vi "to_json.vi"(8 "error in":errorcluster, 11 "target in":refnum<class "target.lvclass">) -> (0 "error out":errorcluster, 2 "json":string, 3 "target out":refnum<class "target.lvclass">, 4 "Not Default":bool)   [LabVIEW 2020, in "datasources.lvlib" / "target.lvclass"]
uses:
  target.lvclass
  target.lvclass/target.ctl
  dataset/dataset.lvclass/dataset.ctl
  92ef1fda-d962-45ff-88fd-c2047d5c0ec4.vi
  9fa72010-cb42-47d4-8643-e7e5955f5446.vi
  d6cf4258-1369-4a0e-93db-dcab189557e5.vi
  b2c1eefe-8312-4a03-882f-d0c7cc634c10.vi
  dataset/datasetName.get.vi
  dataset/datasetDescription.get.vi
  dataset/rid.get.vi
  <vilib>/JDP Science/JSONtext/Variant to JSON Text.vi
  <vilib>/JDP Science/JSONtext/support/Format JSON Object.vi
  <vilib>/JDP Science/JSONtext/LVClass Serializer/JSONtext LVClass Serializer.lvclass
  nominal types/properties/properties.lvclass
  nominal types/labels/labels.lvclass
  nominal types/channelConfig/channelConfig.lvclass
  nominal types/workspace/workspace.lvclass
  <vilib>/JDP Science/JSONtext/JSONtext.lvlib
  dataset/dataset.lvclass
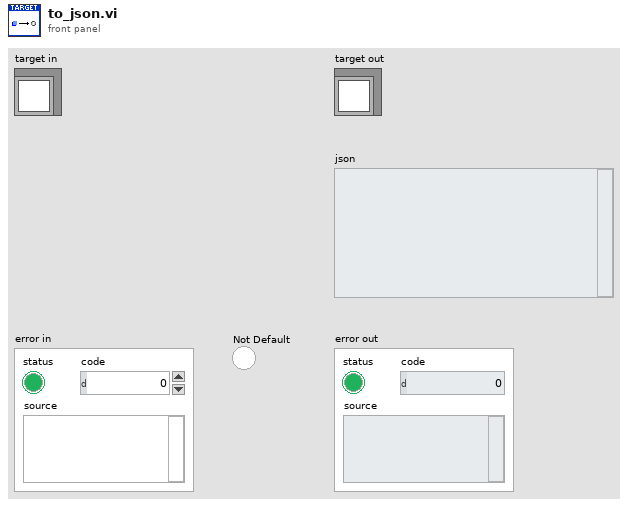
[diagram p1: front panel]
types:
  T1 = cluster{"type":string, "existing":cluster{"datasetRid":string}}
  T2 = cluster{"Accessors:datasetName":string, "Accessors:datasetDescription":string}
  T3 = cluster{"Accessors:datasetName":bool, "Accessors:datasetDescription":bool}
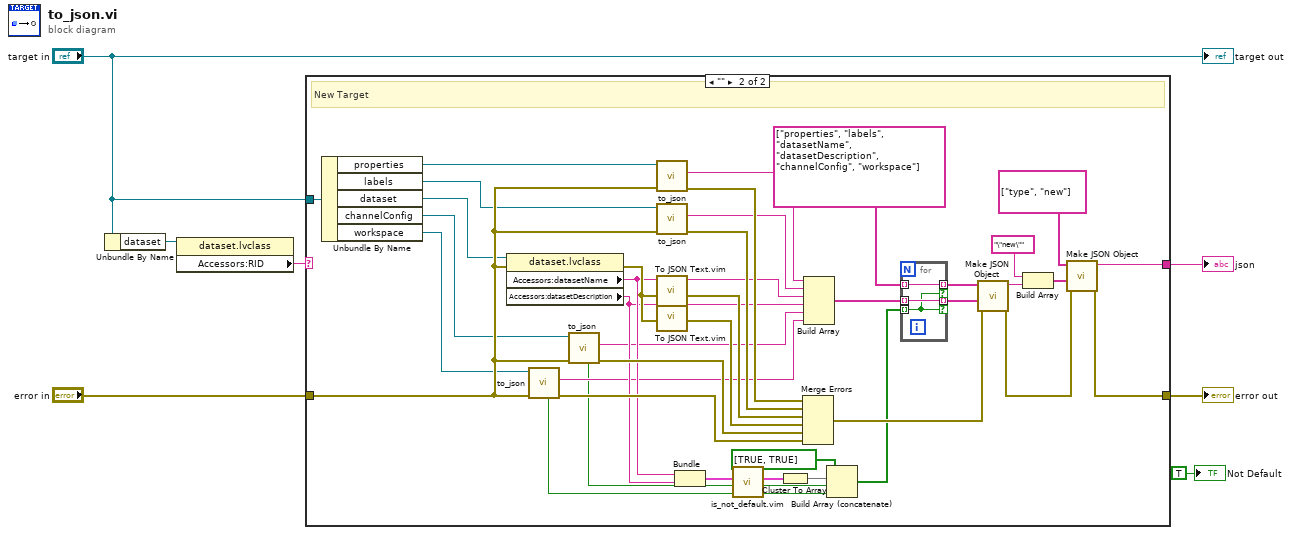
[diagram p0: block diagram]
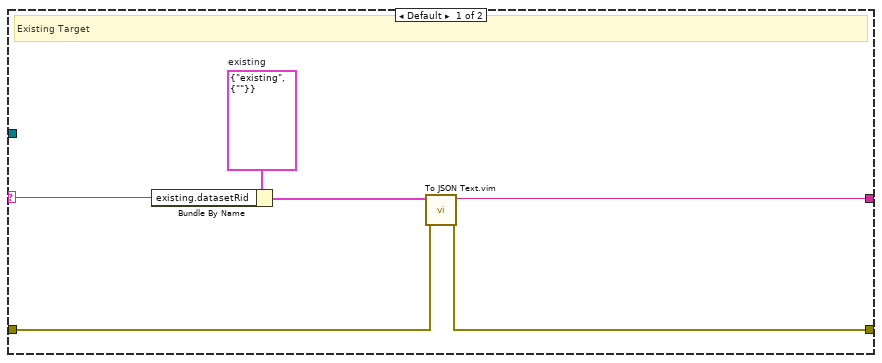
[diagram p2: hidden frame]
diagram:
  n1 = Unbundle By Name("target in") -> ("dataset"=w3:refnum<class "dataset.lvclass">)
  n2 = property class="dataset.lvclass"(reference=w3) -> ("Accessors:RID"=w2:string)  [unwired: 1 in, 2 out]
  n3 = case shown="\"\"" w2 {
    selector: w2 -> [w12 _]
    tunnel: [w10 w34] -> w7
    tunnel: "error in" -> [w9 w53]
    tunnel: [w8 w32] -> w5
    tunnel: "target in" -> [_ w47]
    frame Default {
      w13 = T1 {"type"="existing", "existing"={"datasetRid"=""}}  # existing
      # "Existing Target"
      n4 = Bundle By Name(cluster=w13, "existing.datasetRid"=w12) -> (w11:T1)
      n5 = call "To JSON Text.vim"("error in (no error)"=w9, "Anything"=w11) -> ("error out"=w8:errorcluster, "<JSON>"=w10:string)  [unwired: 8 in]
    }
    frame "" {
      # "New Target"
      n6 = Unbundle By Name(w47) -> ("properties"=w46:refnum<class "properties.lvclass">, "labels"=w45:refnum<class "labels.lvclass">, "dataset"=w27:refnum<class "dataset.lvclass">, "channelConfig"=w26:refnum<class "channelConfig.lvclass">, "workspace"=w25:refnum<class "workspace.lvclass">)
      n7 = property class="dataset.lvclass"(reference=w27, error in=w53) -> (error out=w54:errorcluster, "Accessors:datasetName"=w19:string, "Accessors:datasetDescription"=w18:string)  [unwired: 1 out]
      n8 = call-dynamic "to_json.vi"("error in"=w53, "workspace in"=w25) -> ("error out"=w40:errorcluster, "json"=w16:string, "Not Default"=w14:bool)  [unwired: 6 in, 1 out]
      n9 = call-dynamic "to_json.vi"("error in"=w53, "channelConfig in"=w26) -> ("error out"=w48:errorcluster, "json"=w17:string, "Not Default"=w15:bool)  [unwired: 6 in, 1 out]
      n10 = call-dynamic "to_json.vi"("error in"=w53, "properties in"=w46) -> ("error out"=w52:errorcluster, "json"=w44:string)  [unwired: 6 in, 2 out]
      n11 = call-dynamic "to_json.vi"("error in"=w53, "labels in"=w45) -> ("error out"=w51:errorcluster, "json"=w43:string)  [unwired: 6 in, 2 out]
      n12 = call "To JSON Text.vim"("error in (no error)"=w54, "Anything"=w19) -> ("error out"=w50:errorcluster, "<JSON>"=w42:string)  [unwired: 8 in]
      n13 = call "To JSON Text.vim"("error in (no error)"=w54, "Anything"=w18) -> ("error out"=w49:errorcluster, "<JSON>"=w41:string)  [unwired: 8 in]
      n14 = Bundle("Accessors:datasetName"=w19, "Accessors:datasetDescription"=w18) -> (w24:T2)  [unwired: 1 in]
      n15 = call "is_not_default.vim"("data"=w24) -> ("Not Default"=w23:T3)  [unwired: 10 in]
      n16 = Cluster To Array(cluster=w23) -> (array=w22:bool[])
      n17 = Merge Errors(w52, w51, w50, w49, w48, w40) -> (w39:errorcluster)
      n18 = Build Array(w44, w43, w42, w41, w17, w16) -> (w31:string[])
      n19 = Build Array (concatenate)(bool[] [TRUE, TRUE] ("element"), w22, w15, w14) -> (w20:bool[])
      n20 = for {
        tunnel: w31 -> [w57] mode=indexing
        tunnel: [w57] -> w30 mode=indexing if=w55
        tunnel: string[] ["properties", "labels", "datasetName", "datasetDescription", "channelConfig", "workspace"] ("Item Names") -> [w56] mode=indexing
        tunnel: [w56] -> w28 mode=indexing if=w55
        tunnel: w20 -> [w55] mode=indexing
      }
      n21 = call <vilib>:"Make JSON Object.vi"("error in (no error)"=w39, "JSON Items"=w30, "Item Names"=w28) -> ("error out"=w33:errorcluster, "<JSON>"=w37:string)  [unwired: 7 in]
      n22 = Build Array("\"new\"" ("element"), w37) -> (w35:string[])
      n23 = call <vilib>:"Make JSON Object.vi"("error in (no error)"=w33, "JSON Items"=w35, "Item Names"=string[] ["type", "new"]) -> ("error out"=w32:errorcluster, "<JSON>"=w34:string)  [unwired: 7 in]
    }
  }
  "error out" <- w5
  "json" <- w7
  "target out" <- "target in"
  "Not Default" <- TRUE ("Not Default")
